vi "F710.01.vi"() -> ()   [LabVIEW 2019]
uses:
  <vilib>/Instr/_visa.llb/VISA Open Access Mode.ctl
panel:
  out "status byte":u16
  out "error out":errorcluster
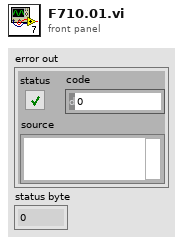
[diagram p1: front panel]
types:
  T1 = typedef "VISA Open Access Mode.ctl" = u32
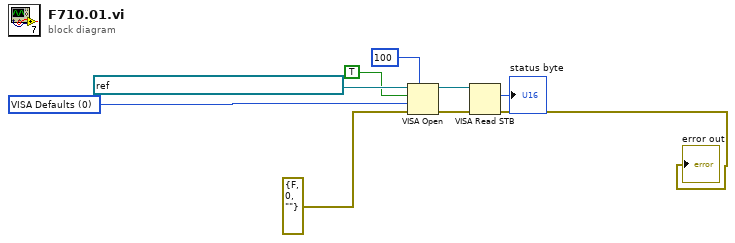
[diagram p0: block diagram]
diagram:
  w6 = T1 0 items=["VISA Defaults"=0, "Exclusive Lock"=1, "Load Configured Settings"=4] ("Access Mode")
  n1 = VISA Open(timeout (0)=u32 100 ("VISA Open timeout (0)"), duplicate session (F)=TRUE, access mode=w6, error in (no error)=errorcluster {"status"=FALSE, "code"=0, "source"=""}, VISA resource name=refnum<visa-resource-name> "USB0::0x046D::0xC21F::B8599589::RAW") -> (VISA resource name=w2:refnum<visa-resource-name>, error out=w3:errorcluster)
  n2 = VISA Read STB(8:w3, 11:w2) -> (0:→"error out":errorcluster, 2:→"status byte":u16)  [unwired: 1 out]
